vi "GetPositionDetails.vi"(9 "Seperator in":string, 10 "Command":string, 11 "Picomotor8752 in":refnum<class "Picomotor8752.lvclass">) -> (1 "RelativeMovement":i32, 2 "DeviceOut":string, 3 "Pico Parameter":T2, 4 "AbsolutePosition":i32, 6 "Position":T1)   [LabVIEW 2013, in "Picomotor8752.lvclass"]
uses:
  Picomotor8752.lvclass
  TypeDefs/ChannelsCluster.ctl
  Picomotor8752.lvclass/Picomotor8752.ctl
  shared/UtilsLib/ClusterManipulation/GetClusterElementByName(String).vi
  shared/UtilsLib/ClusterManipulation/GetClusterElementByName(I32).vi
  ESP301/ESP301.lvclass
  shared/UtilsLib/ClusterManipulation/GetClusterElementByName.lvlib
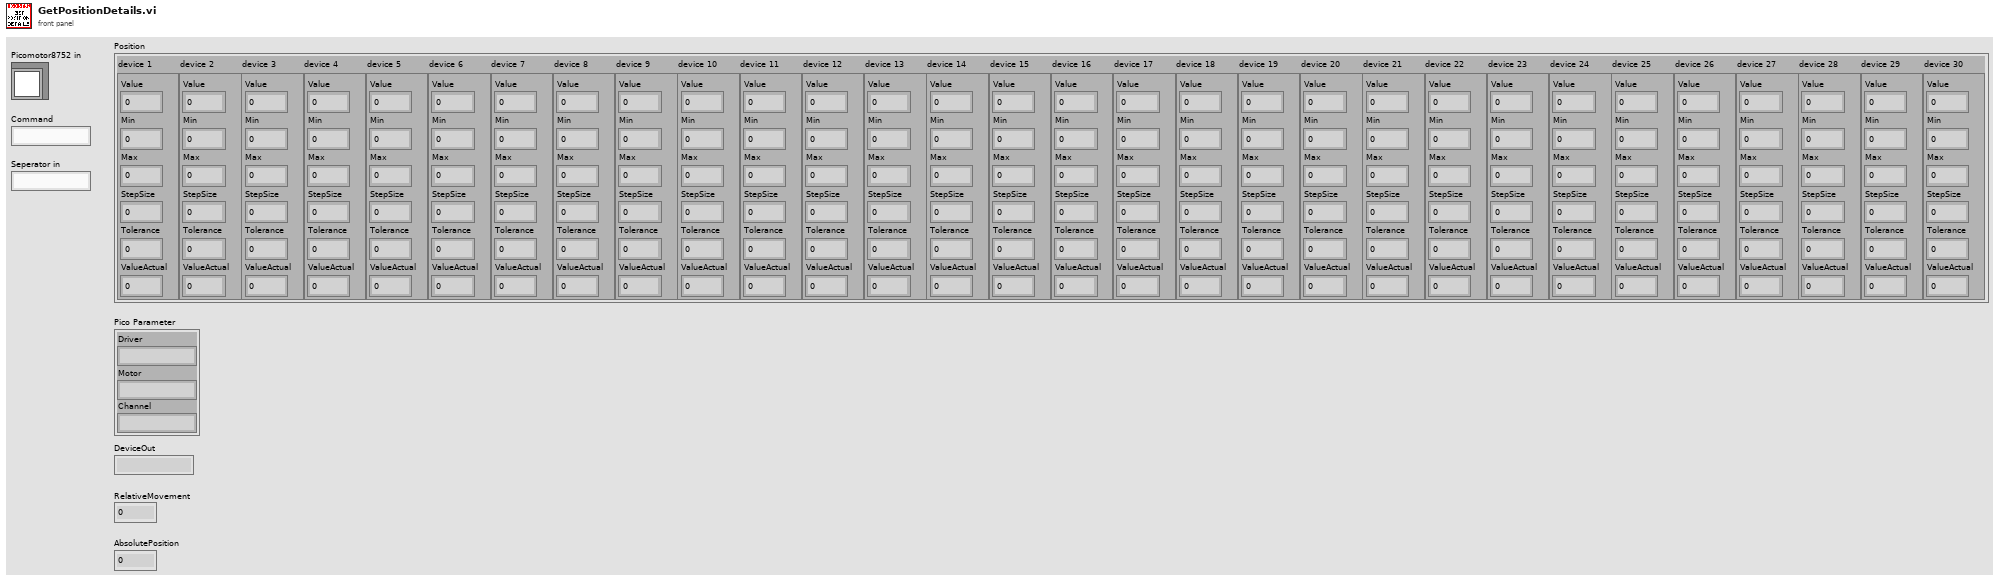
[diagram p1: front panel]
types:
  T1 = typedef "ChannelsCluster.ctl" = cluster{"device 1":cluster{"Value":dbl, "Min":dbl, "Max":dbl, "StepSize":dbl, "Tolerance":dbl, "ValueActual":dbl}, "device 2":cluster{"Value":dbl, "Min":dbl, "Max":dbl, "StepSize":dbl, "Tolerance":dbl, "ValueActual":dbl}, "device 3":cluster{"Value":dbl, "Min":dbl, "Max":dbl, "StepSize":dbl, "Tolerance":dbl, "ValueActual":dbl}, "device 4":cluster{"Value":dbl, "Min":dbl, "Max":dbl, "StepSize":dbl, "Tolerance":dbl, "ValueActual":dbl}, "device 5":cluster{"Value":dbl, "Min":dbl, "Max":dbl, "StepSize":dbl, "Tolerance":dbl, "ValueActual":dbl}, "device 6":cluster{"Value":dbl, "Min":dbl, "Max":dbl, "StepSize":dbl, "Tolerance":dbl, "ValueActual":dbl}, "device 7":cluster{"Value":dbl, "Min":dbl, "Max":dbl, "StepSize":dbl, "Tolerance":dbl, "ValueActual":dbl}, "device 8":cluster{"Value":dbl, "Min":dbl, "Max":dbl, "StepSize":dbl, "Tolerance":dbl, "ValueActual":dbl}, "device 9":cluster{"Value":dbl, "Min":dbl, "Max":dbl, "StepSize":dbl, "Tolerance":dbl, "ValueActual":dbl}, "device 10":cluster{"Value":dbl, "Min":dbl, "Max":dbl, "StepSize":dbl, "Tolerance":dbl, "ValueActual":dbl}, "device 11":cluster{"Value":dbl, "Min":dbl, "Max":dbl, "StepSize":dbl, "Tolerance":dbl, "ValueActual":dbl}, "device 12":cluster{"Value":dbl, "Min":dbl, "Max":dbl, "StepSize":dbl, "Tolerance":dbl, "ValueActual":dbl}, "device 13":cluster{"Value":dbl, "Min":dbl, "Max":dbl, "StepSize":dbl, "Tolerance":dbl, "ValueActual":dbl}, "device 14":cluster{"Value":dbl, "Min":dbl, "Max":dbl, "StepSize":dbl, "Tolerance":dbl, "ValueActual":dbl}, "device 15":cluster{"Value":dbl, "Min":dbl, "Max":dbl, "StepSize":dbl, "Tolerance":dbl, "ValueActual":dbl}, "device 16":cluster{"Value":dbl, "Min":dbl, "Max":dbl, "StepSize":dbl, "Tolerance":dbl, "ValueActual":dbl}, "device 17":cluster{"Value":dbl, "Min":dbl, "Max":dbl, "StepSize":dbl, "Tolerance":dbl, "ValueActual":dbl}, "device 18":cluster{"Value":dbl, "Min":dbl, "Max":dbl, "StepSize":dbl, "Tolerance":dbl, "ValueActual":dbl}, "device 19":cluster{"Value":dbl, "Min":dbl, "Max":dbl, "StepSize":dbl, "Tolerance":dbl, "ValueActual":dbl}, "device 20":cluster{"Value":dbl, "Min":dbl, "Max":dbl, "StepSize":dbl, "Tolerance":dbl, "ValueActual":dbl}, "device 21":cluster{"Value":dbl, "Min":dbl, "Max":dbl, "StepSize":dbl, "Tolerance":dbl, "ValueActual":dbl}, "device 22":cluster{"Value":dbl, "Min":dbl, "Max":dbl, "StepSize":dbl, "Tolerance":dbl, "ValueActual":dbl}, "device 23":cluster{"Value":dbl, "Min":dbl, "Max":dbl, "StepSize":dbl, "Tolerance":dbl, "ValueActual":dbl}, "device 24":cluster{"Value":dbl, "Min":dbl, "Max":dbl, "StepSize":dbl, "Tolerance":dbl, "ValueActual":dbl}, "device 25":cluster{"Value":dbl, "Min":dbl, "Max":dbl, "StepSize":dbl, "Tolerance":dbl, "ValueActual":dbl}, "device 26":cluster{"Value":dbl, "Min":dbl, "Max":dbl, "StepSize":dbl, "Tolerance":dbl, "ValueActual":dbl}, "device 27":cluster{"Value":dbl, "Min":dbl, "Max":dbl, "StepSize":dbl, "Tolerance":dbl, "ValueActual":dbl}, "device 28":cluster{"Value":dbl, "Min":dbl, "Max":dbl, "StepSize":dbl, "Tolerance":dbl, "ValueActual":dbl}, "device 29":cluster{"Value":dbl, "Min":dbl, "Max":dbl, "StepSize":dbl, "Tolerance":dbl, "ValueActual":dbl}, "device 30":cluster{"Value":dbl, "Min":dbl, "Max":dbl, "StepSize":dbl, "Tolerance":dbl, "ValueActual":dbl}}
  T2 = cluster{"Driver":string, "Motor":string, "Channel":string}
  T3 = cluster{"device 1":string, "device 2":string, "device 3":string, "device 4":string, "device 5":string, "device 6":string, "device 7":string, "device 8":string, "device 9":string, "device 10":string, "device 11":string, "device 12":string, "device 13":string, "device 14":string, "device 15":string, "device 16":string, "device 17":string, "device 18":string, "device 19":string, "device 20":string, "device 21":string, "device 22":string, "device 23":string, "device 24":string, "device 25":string, "device 26":string, "device 27":string, "device 28":string, "device 29":string, "device 30":string}
  T4 = cluster{"device 1":cluster{"Value":dbl, "Min":dbl, "Max":dbl, "StepSize":dbl, "Tolerance":dbl, "ValueActual":dbl}, "device 2":cluster{"Value":dbl, "Min":dbl, "Max":dbl, "StepSize":dbl, "Tolerance":dbl, "ValueActual":dbl}, "device 3":cluster{"Value":dbl, "Min":dbl, "Max":dbl, "StepSize":dbl, "Tolerance":dbl, "ValueActual":dbl}, "device 4":cluster{"Value":dbl, "Min":dbl, "Max":dbl, "StepSize":dbl, "Tolerance":dbl, "ValueActual":dbl}, "device 5":cluster{"Value":dbl, "Min":dbl, "Max":dbl, "StepSize":dbl, "Tolerance":dbl, "ValueActual":dbl}, "device 6":cluster{"Value":dbl, "Min":dbl, "Max":dbl, "StepSize":dbl, "Tolerance":dbl, "ValueActual":dbl}, "device 7":cluster{"Value":dbl, "Min":dbl, "Max":dbl, "StepSize":dbl, "Tolerance":dbl, "ValueActual":dbl}, "device 8":cluster{"Value":dbl, "Min":dbl, "Max":dbl, "StepSize":dbl, "Tolerance":dbl, "ValueActual":dbl}, "device 9":cluster{"Value":dbl, "Min":dbl, "Max":dbl, "StepSize":dbl, "Tolerance":dbl, "ValueActual":dbl}, "device 10":cluster{"Value":dbl, "Min":dbl, "Max":dbl, "StepSize":dbl, "Tolerance":dbl, "ValueActual":dbl}, "device 11":cluster{"Value":dbl, "Min":dbl, "Max":dbl, "StepSize":dbl, "Tolerance":dbl, "ValueActual":dbl}, "device 12":cluster{"Value":dbl, "Min":dbl, "Max":dbl, "StepSize":dbl, "Tolerance":dbl, "ValueActual":dbl}, "device 13":cluster{"Value":dbl, "Min":dbl, "Max":dbl, "StepSize":dbl, "Tolerance":dbl, "ValueActual":dbl}, "device 14":cluster{"Value":dbl, "Min":dbl, "Max":dbl, "StepSize":dbl, "Tolerance":dbl, "ValueActual":dbl}, "device 15":cluster{"Value":dbl, "Min":dbl, "Max":dbl, "StepSize":dbl, "Tolerance":dbl, "ValueActual":dbl}, "device 16":cluster{"Value":dbl, "Min":dbl, "Max":dbl, "StepSize":dbl, "Tolerance":dbl, "ValueActual":dbl}, "device 17":cluster{"Value":dbl, "Min":dbl, "Max":dbl, "StepSize":dbl, "Tolerance":dbl, "ValueActual":dbl}, "device 18":cluster{"Value":dbl, "Min":dbl, "Max":dbl, "StepSize":dbl, "Tolerance":dbl, "ValueActual":dbl}, "device 19":cluster{"Value":dbl, "Min":dbl, "Max":dbl, "StepSize":dbl, "Tolerance":dbl, "ValueActual":dbl}, "device 20":cluster{"Value":dbl, "Min":dbl, "Max":dbl, "StepSize":dbl, "Tolerance":dbl, "ValueActual":dbl}, "device 21":cluster{"Value":dbl, "Min":dbl, "Max":dbl, "StepSize":dbl, "Tolerance":dbl, "ValueActual":dbl}, "device 22":cluster{"Value":dbl, "Min":dbl, "Max":dbl, "StepSize":dbl, "Tolerance":dbl, "ValueActual":dbl}, "device 23":cluster{"Value":dbl, "Min":dbl, "Max":dbl, "StepSize":dbl, "Tolerance":dbl, "ValueActual":dbl}, "device 24":cluster{"Value":dbl, "Min":dbl, "Max":dbl, "StepSize":dbl, "Tolerance":dbl, "ValueActual":dbl}, "device 25":cluster{"Value":dbl, "Min":dbl, "Max":dbl, "StepSize":dbl, "Tolerance":dbl, "ValueActual":dbl}, "device 26":cluster{"Value":dbl, "Min":dbl, "Max":dbl, "StepSize":dbl, "Tolerance":dbl, "ValueActual":dbl}, "device 27":cluster{"Value":dbl, "Min":dbl, "Max":dbl, "StepSize":dbl, "Tolerance":dbl, "ValueActual":dbl}, "device 28":cluster{"Value":dbl, "Min":dbl, "Max":dbl, "StepSize":dbl, "Tolerance":dbl, "ValueActual":dbl}, "device 29":cluster{"Value":dbl, "Min":dbl, "Max":dbl, "StepSize":dbl, "Tolerance":dbl, "ValueActual":dbl}, "device 30":cluster{"Value":dbl, "Min":dbl, "Max":dbl, "StepSize":dbl, "Tolerance":dbl, "ValueActual":dbl}}
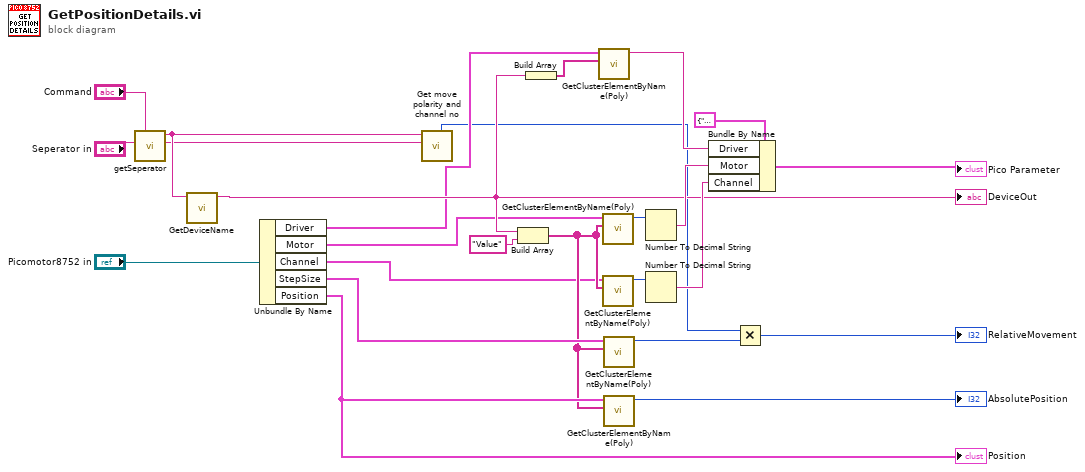
[diagram p0: block diagram]
diagram:
  n1 = call "getSeperator.vi"("Channel Seperator (\"\")"="Seperator in", "Command"="Command") -> ("Channel"=w3:string, "Seperator (e.g. \"Channel1\")"=w5:string)  [unwired: 8 in]
  n2 = call "GetDeviceName.vi"("Seperator (e.g. \"Channel1\")"=w5) -> ("String"=w16:string)  [unwired: 10 in]
  "DeviceOut" <- w16
  n3 = Unbundle By Name("Picomotor8752 in") -> ("Driver"=w14:T3, "Motor"=w8:T4, "Channel"=w10:T4, "StepSize"=w20:T1, "Position"=w19:T1)
  "Position" <- w19
  n4 = call "Get move polarity and channel no.vi"("Channel in"=w3, "Channel string In"=w5) -> ("Numeric"=w6:i32)  [unwired: 7 in, 2 out]
  n5 = Build Array(w16, "Value" ("string")) -> (w18:string[])
  n6 = Build Array(w16) -> (w15:string[])
  n7 = call-poly "GetClusterElementByName(Poly).vi"("ElementName"=w15, "Cluster"=w14) -> ("ValueOut"=w22:string)  [unwired: 8 in, 1 out]
  n8 = call-poly "GetClusterElementByName(Poly).vi"("ElementName"=w18, "Cluster"=w8) -> ("ValueOut"=w9:i32)  [unwired: 8 in, 1 out]
  n9 = call-poly "GetClusterElementByName(Poly).vi"("ElementName"=w18, "Cluster"=w10) -> ("ValueOut"=w11:i32)  [unwired: 8 in, 1 out]
  n10 = call-poly "GetClusterElementByName(Poly).vi"("ElementName"=w18, "Cluster"=w20) -> ("ValueOut"=w12:i32)  [unwired: 8 in, 1 out]
  n11 = call-poly "GetClusterElementByName(Poly).vi"("ElementName"=w18, "Cluster"=w19) -> ("ValueOut"=→"AbsolutePosition":i32)  [unwired: 8 in, 1 out]
  n12 = Number To Decimal String(number=w9) -> (decimal integer string=w23:string)  [unwired: 1 in]
  n13 = Number To Decimal String(number=w11) -> (decimal integer string=w24:string)  [unwired: 1 in]
  n14 = Bundle By Name(cluster=T2 {"Driver"="", "Motor"="", "Channel"=""} ("Pico Parameter"), "Driver"=w22, "Motor"=w23, "Channel"=w24) -> (→"Pico Parameter":T2)
  n15 = Multiply(x=w6, y=w12) -> (x*y=→"RelativeMovement":i32)
